vi "+S2C_PCIe7841_Process.vi"(8 "Error In":errorcluster) -> (0 "Error Out":errorcluster)   [LabVIEW 2015]
uses:
  VIs/Typedefs/S2C_PCIe7841_Type_Conn0.ctl
  VIs/Typedefs/S2C_PCIe7841_Type_Conn1.ctl
  VIs/Typedefs/S2C_PCIe7841_Type_Conn2.ctl
  VIs/Typedefs/S2C_PCIe7841_Type_Conn0Write.ctl
  VIs/Typedefs/S2C_PCIe7841_Type_Conn1Write.ctl
  VIs/Typedefs/S2C_PCIe7841_Type_Conn2Write.ctl
  VIs/S2C_PCIe7841_Proc_Globals.vi
panel:
  out "Init":bool
  out "Err":bool
  in  "Clear":bool
  out "Exit":bool
  in  "LogDepth":u32=10 caption="Log Depth"
  in  "CtrlTab":T1(tab)
  in  "P1":T2={"Conn0"={"Port 0"={"LxfIpapPower"=TRUE, "LxfAinDiffSelect"=FALSE, "LxfSpare"=FALSE, "VlacSafeIntLock"=FALSE, "VlacPosDiffNi"=FALSE, "VlacNegDiffNi"=FALSE, "Audio1"=FALSE, "Audio2"=FALSE, "P0_Send"=FALSE, "P0_Size"=FALSE, "P0_State"=FALSE}, "Port 1"={"Audio3"=TRUE, "PalletId1Bcd1"=FALSE, "PalletId1Bcd2"=FALSE, "PalletId1Bcd4"=FALSE, "PalletId1Bcd8"=FALSE, "PalletId2Bcd1"=FALSE, "PalletId2Bcd2"=FALSE, "PalletIdLoopback"=FALSE, "P1_Send"=FALSE, "P1_Size"=FALSE, "P1_State"=FALSE}, "P1C1Exe"=FALSE}}
  in  "P2":T3={"Conn1"={"Port 0"={"MeasM1ErgInp"=TRUE, "MeasLoadBxAct"=FALSE, "MeasLoadBxNeu"=FALSE, "MeasDiffProbAct"=FALSE, "MeasDiffProbNeu"=FALSE, "MeasRemReturn"=FALSE, "MeasBipReturn"=FALSE, "MeasM2ErgInp"=FALSE, "P3_Send"=FALSE, "P3_Size"=FALSE, "P3_State"=FALSE}, "Port 1"={"MeasBipErgInp"=TRUE, "MeasLxBiM1ErgInp"=FALSE, "MeasLxBipM1Rtn"=FALSE, "MeasLxfLigRtn"=FALSE, "MeasLxfLigErgInp"=FALSE, "MeasGndResRtn"=FALSE, "MeasGndResAct"=FALSE, "MeasHomerRelay"=FALSE, "P1_Send"=FALSE, "P1_Size"=FALSE, "P1_State"=FALSE}, "Port 2"={"RemRelayCtrl1"=TRUE, "RemRelayCtrl2"=FALSE, "RemSpare"=FALSE, "RemLoopback"=FALSE, "Mono1Cut_HS"=FALSE, "Mono1Coag_HS"=FALSE, "Mono1Spare"=FALSE, "Mono1Loopback"=FALSE, "P2_Send"=FALSE, "P2_Size"=FALSE, "P2_State"=FALSE}, "Port 3"={"Mono2Cut_HS"=TRUE, "Mono2Coag_HS"=FALSE, "Mono2Spare"=FALSE, "Mono2Loopback"=FALSE, "SmokeBip_HS"=FALSE, "SmokeEvac2"=FALSE, "SmokeEvac1"=FALSE, "SmokeEvacLB"=FALSE, "P3_Send"=FALSE, "P3_Size"=FALSE, "P3_State"=FALSE}, "Port 4"={"MeasSpare"=TRUE, "MeasHomerRtn"=FALSE, "MeasHomerDrive"=FALSE, "MeasLoopback"=FALSE, "VlacDcPwrEnbl"=FALSE, "VlacUartTxNi"=FALSE, "VlacUartRxNi"=FALSE, "VlacRmtPwrNi"=FALSE, "P4_Send"=FALSE, "P4_Size"=FALSE, "P4_State"=FALSE}, "P2C1Exe"=FALSE}}
  in  "P3":T4={"Conn2"={"Port 0"={"TriMono2Mode"=TRUE, "TriMono2Intsy"=FALSE, "TriSliderCtrl"=FALSE, "TriSliderIntsyAdd"=FALSE, "TriSliderIntsyA1"=FALSE, "TriSliderIntsyA0"=FALSE, "TriMono2Slider3"=FALSE, "TriMono2Slider2"=FALSE, "P0_Send"=FALSE, "P0_Size"=FALSE, "P0_State"=FALSE}, "Port 1"={"TriMono2Slider1"=TRUE, "TriSliderIntsyEnbl"=FALSE, "TriSliderEnbl"=FALSE, "TriSpare"=FALSE, "Free1"=FALSE, "Free2"=FALSE, "Free3"=FALSE, "Free4"=FALSE, "P1_Send"=FALSE, "P1_Size"=FALSE, "P1_State"=FALSE}, "Port 2"={"LxfHsw0Ctrl"=TRUE, "LxfLpapPwr"=FALSE, "LxfHpapEnbl"=FALSE, "LxfS2/L4Select"=FALSE, "LxfD/ASelect"=FALSE, "LxfAIn/OutSelect"=FALSE, "LxfALadPortSel"=FALSE, "LxfS2/L4Do"=FALSE, "P2_Send"=FALSE, "P2_Size"=FALSE, "P2_State"=FALSE}, "Port 3"={"LxfS2/L4Di"=FALSE, "LxfS3/L3Do"=TRUE, "LxfS3/L3Di"=FALSE, "LxfHpapAi"=FALSE, "LxfDEnable"=FALSE, "LxfDA1"=FALSE, "LxfDA0"=FALSE, "LxfUartSelect"=FALSE, "P3_Send"=FALSE, "P3_Size"=FALSE, "P3_State"=FALSE}, "Port 4"={"LxfNegChLoopBk"=TRUE, "LxfPosChLoopBk"=FALSE, "LxfRs485DriveDir"=FALSE, "LxfHsw1Ctrl"=FALSE, "LoadSwitchRsvd1"=FALSE, "LoadSwitchRsvd2"=FALSE, "LoadSwitchRsvd3"=FALSE, "LoadSwitchRsvd4"=FALSE, "P4_Send"=FALSE, "P4_Size"=FALSE, "P4_State"=FALSE}, "P3C1Exe"=FALSE}}
  in  "P4":T5
  in  "P5":T12 {"Digital Write"."Connector" items=["Connector 0", "Connector 1", "Connector 2"]; "Digital Write"."Conn2_Item" items=["TriMono2Mode"=0, "TriMono2Intsy"=1, "TriSliderCtrl"=2, "TriSliderIntsyAdd"=3, "TriSliderIntsyA1"=4, "TriSliderIntsyA0"=5, "TriMono2Slider3"=6, "TriMono2Slider2"=7, "TriMono2Slider1"=8, "TriSliderIntsyEnbl"=9, "TriSliderEnbl"=10, "TriSpare"=11, "Free1"=12, "Free2"=13, "Free3"=14, "Free4"=15, "LxfHsw0Ctrl"=16, "LxfLpapPwr"=17, "LxfHpapEnbl"=18, "LxfS2/L4Select"=19, "LxfD/ASelect"=20, "LxfAIn/OutSelect"=21, "LxfALadPortSel"=22, "LxfS2/L4Do"=23, "LxfS3/L3Do"=25, "LxfHpapAi"=27, "LxfDEnable"=28, "LxfDA1"=29, "LxfDA0"=30, "LxfUartSelect"=31, "LxfNegChLoopBk"=32, "LxfPosChLoopBk"=33, "LxfRs485DriveDir"=34, "LxfHsw1Ctrl"=35, "LoadSwitchRsvd1"=36, "LoadSwitchRsvd2"=37, "LoadSwitchRsvd3"=38, "LoadSwitchRsvd4"=39]; "Digital Write"."Conn1_Item" items=["MeasM1ErgInput"=0, "MeasLoadBxAct"=1, "MeasLoadBxNeu"=2, "MeasDiffProbAct"=3, "MeasDiffProbNeu"=4, "MeasRemReturn"=5, "MeasBipReturn"=6, "MeasM2ErgInp"=7, "MeasBipErgInp"=8, "MeasLxBpM1ErgInp"=9, "MeasLxBipM1Rtn"=10, "MeasLxfLigRtn"=11, "MeasLxfLigErgInp"=12, "MeasGndResRtn"=13, "MeasGndResAct"=14, "MeasHomerRelay"=15, "RemRelayCtrl1"=16, "RemRelayCtrl2"=17, "RemSpare"=18, "Mono1Cut_HS"=20, "Mono1Coag_HS"=21, "Mono1Spare"=22, "Mono2Cut_HS"=24, "Mono2Coag_HS"=25, "Mono2Spare"=26, "SmokeBip_HS"=28, "MeasSpare"=32, "MeasHomerRtn"=33, "VlacDcPwrEnbl"=36, "VlacUartTxNi"=37]; "Digital Write"."Conn0_Item" items=["LxfIpapPower"=0, "LxfAinDiffSelect"=1, "LxfSpare"=2, "Audio1"=6, "Audio2"=7, "Audio3"=8]; "Digital Read"."Connector" items=["Connector 0", "Connector 1", "Connector 2"]; "Digital Read"."Conn2_Item" items=["TriMono2Mode", "TriMono2Intsy", "TriSliderCtrl", "TriSliderIntsyAdd", "TriSliderIntsyA1", "TriSliderIntsyA0", "TriMono2Slider3", "TriMono2Slider2", "TriMono2Slider1", "TriSliderIntsyEnbl", "TriSliderEnbl", "TriSpare", "Free1", "Free2", "Free3", "Free4", "LxfHsw0Ctrl", "LxfLpapPwr", "LxfHpapEnbl", "LxfS2/L4Select", "LxfD/ASelect", "LxfAIn/OutSelect", "LxfALadPortSel", "LxfS2/L4Do", "LxfS2/L4Di", "LxfS3/L3Do", "LxfS3/L3Di", "LxfHpapAi", "LxfDEnable", "LxfDA1", "LxfDA0", "LxfUartSelect", "LxfNegChLoopBk", "LxfPosChLoopBk", "LxfRs485DriveDir", "LxfHsw1Ctrl", "LoadSwitchRsvd1", "LoadSwitchRsvd2", "LoadSwitchRsvd3", "LoadSwitchRsvd4"]; "Digital Read"."Conn1_Item" items=["MeasM1ErgInput (75kHz)", "MeasLoadBxAct (75kHz)", "MeasLoadBxNeu (75kHz)", "MeasDiffProbAct (75kHz)", "MeasDiffProbNeu (75kHz)", "MeasRemReturn (75kHz)", "MeasBipReturn (75kHz)", "MeasM2ErgInp (75kHz)", "MeasBipErgInp (75kHz)", "MeasLxBpM1ErgInp (75kHz)", "MeasLxBipM1Rtn (75kHz)", "MeasLxfLigRtn (75kHz)", "MeasLxfLigErgInp (75kHz)", "MeasGndResRtn (75kHz)", "MeasGndResAct (75kHz)", "MeasHomerRelay (75kHz)", "RemRelayCtrl1 (75kHz)", "RemRelayCtrl2 (75kHz)", "RemSpare", "RemLoopback", "Mono1Cut_HS (75kHz)", "Mono1Coag_HS (75kHz)", "Mono1Spare", "Mono1Loopback", "Mono2Cut_HS (75kHz)", "Mono2Coag_HS (75kHz)", "Mono2Spare", "Mono2Loopback", "SmokeBip_HS", "SmokeEvac2", "SmokeEvac1", "SmokeEvacLB", "MeasSpare", "MeasHomerRtn", "MeasHomerDrive", "MeasLoopback", "VlacDcPwrEnbl", "VlacUartTxNi", "VlacUartRxNi", "VlacTmtPwrNi"]; "Digital Read"."Conn0_Item" items=["LxfIpapPower", "LxfAinDiffSelect", "LxfSpare", "VlacSafeIntLock", "VlacPosDiffNi", "VlacNegDiffNi", "Audio1", "Audio2", "Audio3", "PalletId1BCD1", "PalletId1BCD2", "PalletId1BCD4", "PalletId1BCD8", "PalletId2BCD1", "PalletId2BCD2", "PalletIdLoopback"]}
  in  "P6":T13 {"Analog Read"."AO7" min=-10.0 max=10.0 format="%#.6g"; "Analog Read"."AO6" min=-10.0 max=10.0 format="%#.6g"; "Analog Read"."AO5" min=-10.0 max=10.0 format="%#.6g"; "Analog Read"."AO4" min=-10.0 max=10.0 format="%#.6g"; "Analog Read"."AO3" min=-10.0 max=10.0 format="%#.6g"; "Analog Read"."AO2" min=-10.0 max=10.0 format="%#.6g"; "Analog Read"."AO1" min=-10.0 max=10.0 format="%#.6g"; "Analog Read"."AO0" min=-10.0 max=10.0 format="%#.6g"; "Analog Read"."AI7" min=-10.0 max=10.0 format="%#.6g"; "Analog Read"."AI6" min=-10.0 max=10.0 format="%#.6g"; "Analog Read"."AI5" min=-10.0 max=10.0 format="%#.6g"; "Analog Read"."AI4" min=-10.0 max=10.0 format="%#.6g"; "Analog Read"."AI3" min=-10.0 max=10.0 format="%#.6g"; "Analog Read"."AI2" min=-10.0 max=10.0 format="%#.6g"; "Analog Read"."AI1" min=-10.0 max=10.0 format="%#.6g"; "Analog Read"."AI0" min=-10.0 max=10.0 format="%#.6g"; "Analog Write"."AO7" min=-10.0 max=10.0 format="%#.6g"; "Analog Write"."AO6" min=-10.0 max=10.0 format="%#.6g"; "Analog Write"."AO5" min=-10.0 max=10.0 format="%#.6g"; "Analog Write"."AO4" min=-10.0 max=10.0 format="%#.6g"; "Analog Write"."AO3" min=-10.0 max=10.0 format="%#.6g"; "Analog Write"."AO2" min=-10.0 max=10.0 format="%#.6g"; "Analog Write"."AO1" min=-10.0 max=10.0 format="%#.6g"; "Analog Write"."AO0" min=-10.0 max=10.0 format="%#.6g"}
  in  "CommLog":string caption="Communication Log"
  # "Main Cluster:\n394x886\n1 = 355x876\n2 = 355x438\n3 = 355x292\n4 = 163x438\n6 = 163x292\n8 = 163x219"
  # "PCIe7841 Driver Panel"
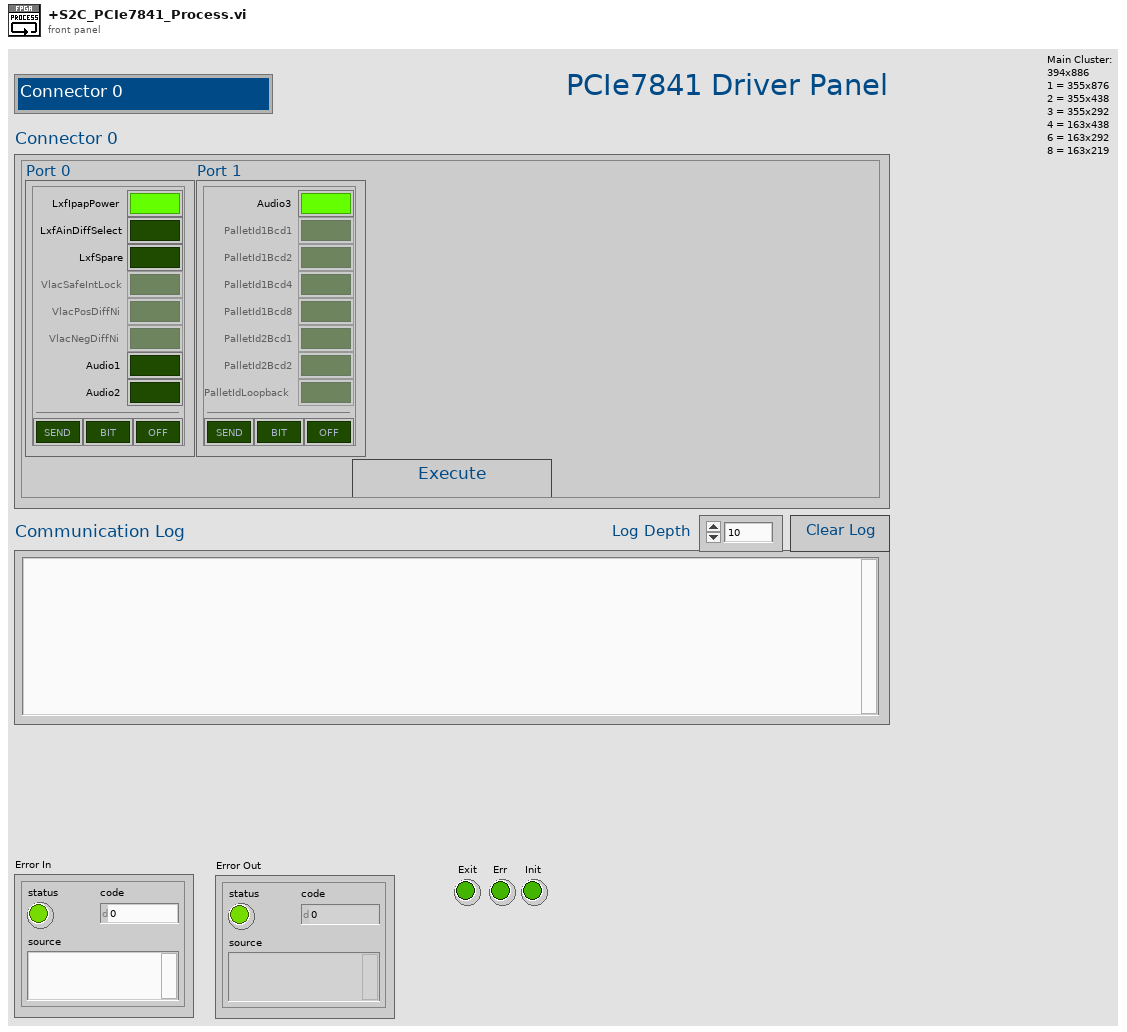
[diagram p1: front panel]
types:
  T1 = enum32{"Connector 0", "Connector 1", "Connector 2", "Status", "Digital IO", "Analog IO"}
  T2 = cluster{"Conn0":cluster{"Port 0":cluster{"LxfIpapPower":bool, "LxfAinDiffSelect":bool, "LxfSpare":bool, "VlacSafeIntLock":bool, "VlacPosDiffNi":bool, "VlacNegDiffNi":bool, "Audio1":bool, "Audio2":bool, "P0_Send":bool, "P0_Size":bool, "P0_State":bool}, "Port 1":cluster{"Audio3":bool, "PalletId1Bcd1":bool, "PalletId1Bcd2":bool, "PalletId1Bcd4":bool, "PalletId1Bcd8":bool, "PalletId2Bcd1":bool, "PalletId2Bcd2":bool, "PalletIdLoopback":bool, "P1_Send":bool, "P1_Size":bool, "P1_State":bool}, "P1C1Exe":bool}}
  T3 = cluster{"Conn1":cluster{"Port 0":cluster{"MeasM1ErgInp":bool, "MeasLoadBxAct":bool, "MeasLoadBxNeu":bool, "MeasDiffProbAct":bool, "MeasDiffProbNeu":bool, "MeasRemReturn":bool, "MeasBipReturn":bool, "MeasM2ErgInp":bool, "P3_Send":bool, "P3_Size":bool, "P3_State":bool}, "Port 1":cluster{"MeasBipErgInp":bool, "MeasLxBiM1ErgInp":bool, "MeasLxBipM1Rtn":bool, "MeasLxfLigRtn":bool, "MeasLxfLigErgInp":bool, "MeasGndResRtn":bool, "MeasGndResAct":bool, "MeasHomerRelay":bool, "P1_Send":bool, "P1_Size":bool, "P1_State":bool}, "Port 2":cluster{"RemRelayCtrl1":bool, "RemRelayCtrl2":bool, "RemSpare":bool, "RemLoopback":bool, "Mono1Cut_HS":bool, "Mono1Coag_HS":bool, "Mono1Spare":bool, "Mono1Loopback":bool, "P2_Send":bool, "P2_Size":bool, "P2_State":bool}, "Port 3":cluster{"Mono2Cut_HS":bool, "Mono2Coag_HS":bool, "Mono2Spare":bool, "Mono2Loopback":bool, "SmokeBip_HS":bool, "SmokeEvac2":bool, "SmokeEvac1":bool, "SmokeEvacLB":bool, "P3_Send":bool, "P3_Size":bool, "P3_State":bool}, "Port 4":cluster{"MeasSpare":bool, "MeasHomerRtn":bool, "MeasHomerDrive":bool, "MeasLoopback":bool, "VlacDcPwrEnbl":bool, "VlacUartTxNi":bool, "VlacUartRxNi":bool, "VlacRmtPwrNi":bool, "P4_Send":bool, "P4_Size":bool, "P4_State":bool}, "P2C1Exe":bool}}
  T4 = cluster{"Conn2":cluster{"Port 0":cluster{"TriMono2Mode":bool, "TriMono2Intsy":bool, "TriSliderCtrl":bool, "TriSliderIntsyAdd":bool, "TriSliderIntsyA1":bool, "TriSliderIntsyA0":bool, "TriMono2Slider3":bool, "TriMono2Slider2":bool, "P0_Send":bool, "P0_Size":bool, "P0_State":bool}, "Port 1":cluster{"TriMono2Slider1":bool, "TriSliderIntsyEnbl":bool, "TriSliderEnbl":bool, "TriSpare":bool, "Free1":bool, "Free2":bool, "Free3":bool, "Free4":bool, "P1_Send":bool, "P1_Size":bool, "P1_State":bool}, "Port 2":cluster{"LxfHsw0Ctrl":bool, "LxfLpapPwr":bool, "LxfHpapEnbl":bool, "LxfS2/L4Select":bool, "LxfD/ASelect":bool, "LxfAIn/OutSelect":bool, "LxfALadPortSel":bool, "LxfS2/L4Do":bool, "P2_Send":bool, "P2_Size":bool, "P2_State":bool}, "Port 3":cluster{"LxfS2/L4Di":bool, "LxfS3/L3Do":bool, "LxfS3/L3Di":bool, "LxfHpapAi":bool, "LxfDEnable":bool, "LxfDA1":bool, "LxfDA0":bool, "LxfUartSelect":bool, "P3_Send":bool, "P3_Size":bool, "P3_State":bool}, "Port 4":cluster{"LxfNegChLoopBk":bool, "LxfPosChLoopBk":bool, "LxfRs485DriveDir":bool, "LxfHsw1Ctrl":bool, "LoadSwitchRsvd1":bool, "LoadSwitchRsvd2":bool, "LoadSwitchRsvd3":bool, "LoadSwitchRsvd4":bool, "P4_Send":bool, "P4_Size":bool, "P4_State":bool}, "P3C1Exe":bool}}
  T5 = cluster{"Status":cluster{"P4C1Exe":bool, "Stat0":cluster{"Port 0":cluster{"B0":bool, "B1":bool, "B2":bool, "B3":bool, "B4":bool, "B5":bool, "B6":bool, "B7":bool}, "Port 1":cluster{"B0":bool, "B1":bool, "B2":bool, "B3":bool, "B4":bool, "B5":bool, "B6":bool, "B7":bool}}, "Stat1":cluster{"Port 0":cluster{"B0":bool, "B1":bool, "B2":bool, "B3":bool, "B4":bool, "B5":bool, "B6":bool, "B7":bool}, "Port 1":cluster{"B0":bool, "B1":bool, "B2":bool, "B3":bool, "B4":bool, "B5":bool, "B6":bool, "B7":bool}, "Port 2":cluster{"B0":bool, "B1":bool, "B2":bool, "B3":bool, "B4":bool, "B5":bool, "B6":bool, "B7":bool}, "Port 3":cluster{"B0":bool, "B1":bool, "B2":bool, "B3":bool, "B4":bool, "B5":bool, "B6":bool, "B7":bool}, "Port 4":cluster{"B0":bool, "B1":bool, "B2":bool, "B3":bool, "B4":bool, "B5":bool, "B6":bool, "B7":bool}}, "Stat2":cluster{"Port 0":cluster{"B0":bool, "B1":bool, "B2":bool, "B3":bool, "B4":bool, "B5":bool, "B6":bool, "B7":bool}, "Port 1":cluster{"B0":bool, "B1":bool, "B2":bool, "B3":bool, "B4":bool, "B5":bool, "B6":bool, "B7":bool}, "Port 2":cluster{"B0":bool, "B1":bool, "B2":bool, "B3":bool, "B4":bool, "B5":bool, "B6":bool, "B7":bool}, "Port 3":cluster{"B0":bool, "B1":bool, "B2":bool, "B3":bool, "B4":bool, "B5":bool, "B6":bool, "B7":bool}, "Port 4":cluster{"B0":bool, "B1":bool, "B2":bool, "B3":bool, "B4":bool, "B5":bool, "B6":bool, "B7":bool}}}}
  T6 = typedef "S2C_PCIe7841_Type_Conn0.ctl" = u16
  T7 = typedef "S2C_PCIe7841_Type_Conn1.ctl" = u16
  T8 = typedef "S2C_PCIe7841_Type_Conn2.ctl" = u16
  T9 = typedef "S2C_PCIe7841_Type_Conn0Write.ctl" = u16
  T10 = typedef "S2C_PCIe7841_Type_Conn1Write.ctl" = u16
  T11 = typedef "S2C_PCIe7841_Type_Conn2Write.ctl" = u16
  T12 = cluster{"Digital Read":cluster{"P5C2Exe":bool, "Conn0_Item":T6, "Conn1_Item":T7, "Conn2_Item":T8, "Connector":u16, "StateOut":bool}, "Digital Write":cluster{"Connector":u16, "Conn0_Item":T9, "Conn1_Item":T10, "Conn2_Item":T11, "StateIn":bool, "P5C1Exe":bool}}
  T13 = cluster{"Analog Write":cluster{"AO0":dbl, "AO0_Send":bool, "AO1":dbl, "AO1_Send":bool, "AO2":dbl, "AO2_Send":bool, "AO3":dbl, "AO3_Send":bool, "AO4":dbl, "AO4_Send":bool, "AO5":dbl, "AO5_Send":bool, "AO6":dbl, "AO6_Send":bool, "AO7":dbl, "AO7_Send":bool, "P6C1Exe":bool}, "Analog Read":cluster{"AI0":dbl, "AI1":dbl, "AI2":dbl, "AI3":dbl, "AI4":dbl, "AI5":dbl, "AI6":dbl, "AI7":dbl, "AO0":dbl, "AO1":dbl, "AO2":dbl, "AO3":dbl, "AO4":dbl, "AO5":dbl, "AO6":dbl, "AO7":dbl, "P6C2Exe":bool}}
  T14 = cluster{"Caller-Q":refnum<queue>, "Command":string, "Return":string, "Data":variant, "Timeout":dbl}
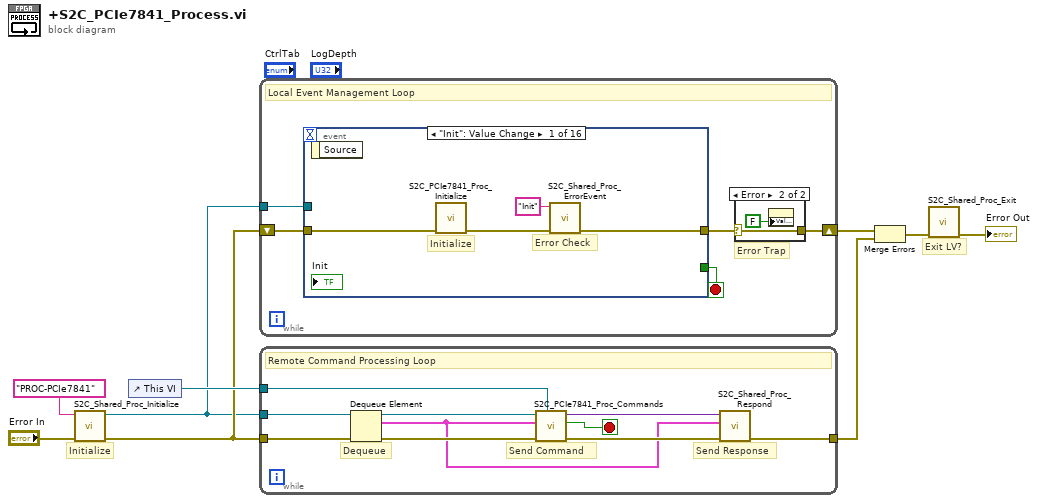
[diagram p0: block diagram]
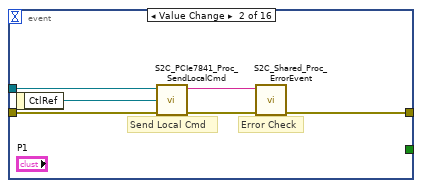
[diagram p3: hidden frame]
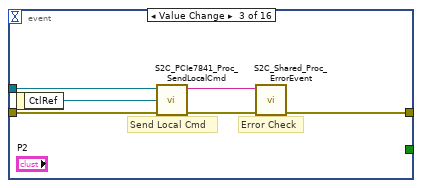
[diagram p4: hidden frame]
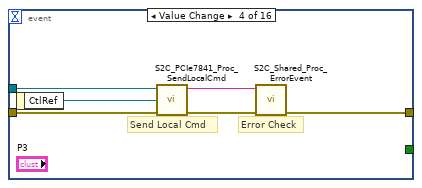
[diagram p5: hidden frame]
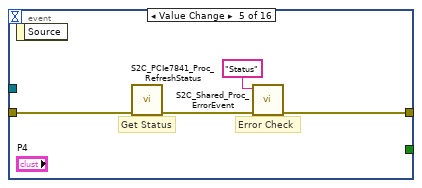
[diagram p6: hidden frame]
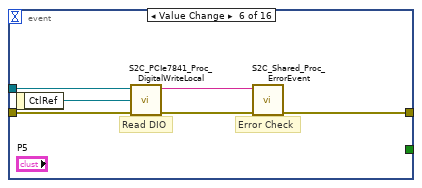
[diagram p7: hidden frame]
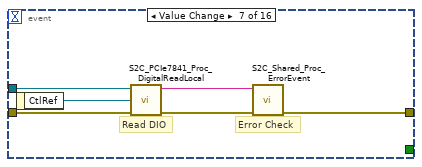
[diagram p8: hidden frame]
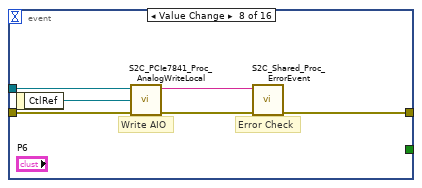
[diagram p9: hidden frame]
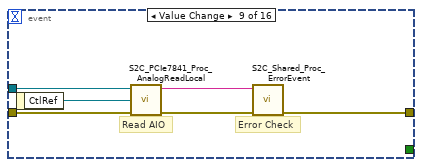
[diagram p10: hidden frame]
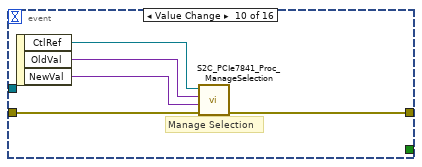
[diagram p11: hidden frame]
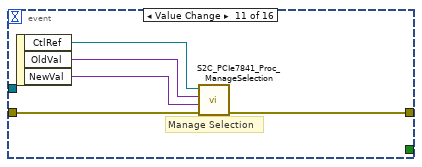
[diagram p12: hidden frame]
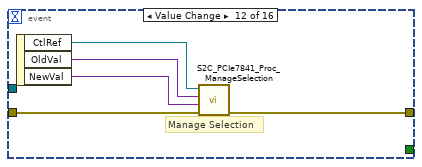
[diagram p13: hidden frame]
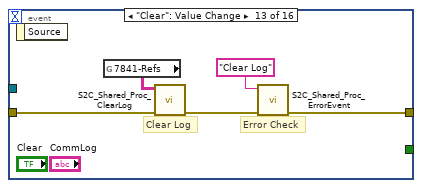
[diagram p14: hidden frame]
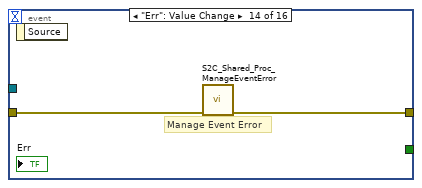
[diagram p15: hidden frame]
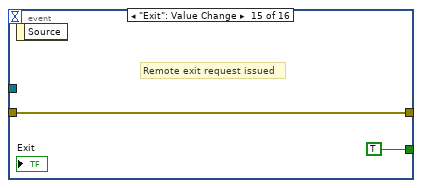
[diagram p16: hidden frame]
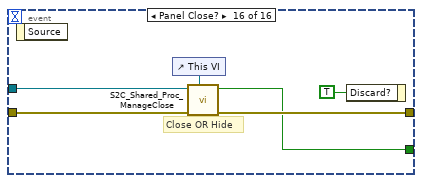
[diagram p17: hidden frame]
diagram:
  # "Exit LV?"
  # "Initialize"
  n1 = call "S2C_Shared_Proc_Initialize.vi"("Error In"="Error In", "Q-Name"="PROC-PCIe7841" ("name (unnamed)")) -> ("Error Out"=w4:errorcluster, "Q-Ref"=w1:refnum<queue>)  [unwired: 8 in]
  n2 = control-ref of="This VI"() -> (w5:refnum<vi>)
  n3 = while {
    tunnel: w1 -> [w13]
    shift-right: [w10] -> w7
    shift-left: w4 -> [w14]
    stop <- w12 stop-if-true
    # "Error Trap"
    # "Local Event Management Loop"
    n4 = event shown="[0] \"Init\": Value Change" {
      selector: _ -> [_ _ _ _ _ _ _ _ _ _ _ _ _ _ _ _]
      dyn-events: _ -> [_ _ _ _ _ _ _ _ _ _ _ _ _ _ _ _]
      timeout: _ -> [_ _ _ _ _ _ _ _ _ _ _ _ _ _ _ _]
      tunnel: w14 -> [w21 w27 w33 w39 w42 w48 w54 w60 w66 w71 w76 w81 w87 w89 w91 w96]
      tunnel: w13 -> [_ w26 w32 w38 _ w46 w52 w58 w64 _ _ _ _ _ _ w94]
      tunnel: [w18 w23 w29 w35 w43 w49 w55 w61 w67 w72 w77 w82 w85 w88 w91 w95] -> w11
      tunnel: [_ _ _ _ _ _ _ _ _ _ _ _ _ _ TRUE ("Discard?") w93] -> w12
      event "Init": Value Change {
        # "Error Check"
        # "Initialize"
        n5 = event-data() -> ()  [unwired: 1 in, 1 out]
        n6 = call "S2C_PCIe7841_Proc_Initialize.vi"("Error In"=w21) -> ("Error Out"=w19:errorcluster)  [unwired: 10 in]
        n7 = call "S2C_Shared_Proc_ErrorEvent.vi"("Error In"=w19, "Command"="Init") -> ("Error Out"=w18:errorcluster)  [unwired: 9 in]
      }
      event "P1.Conn0.P1C1Exe": Value Change {
        # "Error Check"
        # "Send Local Cmd"
        n8 = event-data() -> ("CtlRef"=w25:refnum<vi>)  [unwired: 1 in]
        n9 = call "S2C_PCIe7841_Proc_SendLocalCmd.vi"("Error In"=w27, "ExeRef"=w25, "Q-Ref"=w26) -> ("Error Out"=w24:errorcluster, "Command"=w22:string)  [unwired: 7 in]
        n10 = call "S2C_Shared_Proc_ErrorEvent.vi"("Error In"=w24, "Command"=w22) -> ("Error Out"=w23:errorcluster)  [unwired: 9 in]
      }
      event "P2.Conn1.P2C1Exe": Value Change {
        # "Error Check"
        # "Send Local Cmd"
        n11 = event-data() -> ("CtlRef"=w31:refnum<vi>)  [unwired: 1 in]
        n12 = call "S2C_PCIe7841_Proc_SendLocalCmd.vi"("Error In"=w33, "ExeRef"=w31, "Q-Ref"=w32) -> ("Error Out"=w30:errorcluster, "Command"=w28:string)  [unwired: 7 in]
        n13 = call "S2C_Shared_Proc_ErrorEvent.vi"("Error In"=w30, "Command"=w28) -> ("Error Out"=w29:errorcluster)  [unwired: 9 in]
      }
      event "P3.Conn2.P3C1Exe": Value Change {
        # "Error Check"
        # "Send Local Cmd"
        n14 = event-data() -> ("CtlRef"=w37:refnum<vi>)  [unwired: 1 in]
        n15 = call "S2C_PCIe7841_Proc_SendLocalCmd.vi"("Error In"=w39, "ExeRef"=w37, "Q-Ref"=w38) -> ("Error Out"=w36:errorcluster, "Command"=w34:string)  [unwired: 7 in]
        n16 = call "S2C_Shared_Proc_ErrorEvent.vi"("Error In"=w36, "Command"=w34) -> ("Error Out"=w35:errorcluster)  [unwired: 9 in]
      }
      event "P4.Status.P4C1Exe": Value Change {
        # "Get Status"
        # "Error Check"
        n17 = event-data() -> ()  [unwired: 1 in, 1 out]
        n18 = call "S2C_PCIe7841_Proc_RefreshStatus.vi"("Error In"=w42) -> ("Error Out"=w41:errorcluster)  [unwired: 10 in]
        n19 = call "S2C_Shared_Proc_ErrorEvent.vi"("Error In"=w41, "Command"="Status") -> ("Error Out"=w43:errorcluster)  [unwired: 9 in]
      }
      event "P5.Digital Write.P5C1Exe": Value Change {
        # "Read DIO"
        # "Error Check"
        n20 = event-data() -> ("CtlRef"=w45:refnum<vi>)  [unwired: 1 in]
        n21 = call "S2C_PCIe7841_Proc_DigitalWriteLocal.vi"("Error In"=w48, "ExeRef"=w45, "Q-Ref"=w46) -> ("Error Out"=w47:errorcluster, "Command"=w44:string)  [unwired: 7 in]
        n22 = call "S2C_Shared_Proc_ErrorEvent.vi"("Error In"=w47, "Command"=w44) -> ("Error Out"=w49:errorcluster)  [unwired: 9 in]
      }
      event "P5.Digital Read.P5C2Exe": Value Change {
        # "Read DIO"
        # "Error Check"
        n23 = event-data() -> ("CtlRef"=w51:refnum<vi>)  [unwired: 1 in]
        n24 = call "S2C_PCIe7841_Proc_DigitalReadLocal.vi"("Error In"=w54, "ExeRef"=w51, "Q-Ref"=w52) -> ("Error Out"=w53:errorcluster, "Command"=w50:string)  [unwired: 7 in]
        n25 = call "S2C_Shared_Proc_ErrorEvent.vi"("Error In"=w53, "Command"=w50) -> ("Error Out"=w55:errorcluster)  [unwired: 9 in]
      }
      event "P6.Analog Write.P6C1Exe": Value Change {
        # "Write AIO"
        # "Error Check"
        n26 = event-data() -> ("CtlRef"=w57:refnum<vi>)  [unwired: 1 in]
        n27 = call "S2C_PCIe7841_Proc_AnalogWriteLocal.vi"("Error In"=w60, "ExeRef"=w57, "Q-Ref"=w58) -> ("Error Out"=w59:errorcluster, "Command"=w56:string)  [unwired: 7 in]
        n28 = call "S2C_Shared_Proc_ErrorEvent.vi"("Error In"=w59, "Command"=w56) -> ("Error Out"=w61:errorcluster)  [unwired: 9 in]
      }
      event "P6.Analog Read.P6C2Exe": Value Change {
        # "Read AIO"
        # "Error Check"
        n29 = event-data() -> ("CtlRef"=w63:refnum<vi>)  [unwired: 1 in]
        n30 = call "S2C_PCIe7841_Proc_AnalogReadLocal.vi"("Error In"=w66, "ExeRef"=w63, "Q-Ref"=w64) -> ("Error Out"=w65:errorcluster, "Command"=w62:string)  [unwired: 7 in]
        n31 = call "S2C_Shared_Proc_ErrorEvent.vi"("Error In"=w65, "Command"=w62) -> ("Error Out"=w67:errorcluster)  [unwired: 9 in]
      }
      event "P1.Conn0.Port 0", "P1.Conn0.Port 1": Value Change {
        # "Manage Selection"
        n32 = event-data() -> ("CtlRef"=w68:refnum<vi>, "OldVal"=w69:variant, "NewVal"=w70:variant)  [unwired: 1 in]
        n33 = call "S2C_PCIe7841_Proc_ManageSelection.vi"("Error In"=w71, "NewValue"=w70, "OldValue"=w69, "CtlRef"=w68) -> ("Error Out"=w72:errorcluster)  [unwired: 7 in]
      }
      event "P2.Conn1.Port 0", "P2.Conn1.Port 1", "P2.Conn1.Port 2", "P2.Conn1.Port 3", "P2.Conn1.Port 4": Value Change {
        # "Manage Selection"
        n34 = event-data() -> ("CtlRef"=w73:refnum<vi>, "OldVal"=w74:variant, "NewVal"=w75:variant)  [unwired: 1 in]
        n35 = call "S2C_PCIe7841_Proc_ManageSelection.vi"("Error In"=w76, "NewValue"=w75, "OldValue"=w74, "CtlRef"=w73) -> ("Error Out"=w77:errorcluster)  [unwired: 7 in]
      }
      event "P3.Conn2.Port 0", "P3.Conn2.Port 1", "P3.Conn2.Port 2", "P3.Conn2.Port 3", "P3.Conn2.Port 4": Value Change {
        # "Manage Selection"
        n36 = event-data() -> ("CtlRef"=w78:refnum<vi>, "OldVal"=w79:variant, "NewVal"=w80:variant)  [unwired: 1 in]
        n37 = call "S2C_PCIe7841_Proc_ManageSelection.vi"("Error In"=w81, "NewValue"=w80, "OldValue"=w79, "CtlRef"=w78) -> ("Error Out"=w82:errorcluster)  [unwired: 7 in]
      }
      event "Clear": Value Change {
        # "Error Check"
        # "Clear Log"
        n38 = event-data() -> ()  [unwired: 1 in, 1 out]
        n39 = global read "S2C_PCIe7841_Proc_Globals.vi" "7841-Refs"() -> (w83:string[][])
        n40 = call "S2C_Shared_Proc_ClearLog.vi"("Error In"=w87, "Refs"=w83) -> ("Error Out"=w86:errorcluster)  [unwired: 9 in]
        n41 = call "S2C_Shared_Proc_ErrorEvent.vi"("Error In"=w86, "Command"="Clear Log") -> ("Error Out"=w85:errorcluster)  [unwired: 9 in]
      }
      event "Err": Value Change {
        # "Manage Event Error"
        n42 = event-data() -> ()  [unwired: 1 in, 1 out]
        n43 = call "S2C_Shared_Proc_ManageEventError.vi"("Error In"=w89) -> ("Error Out"=w88:errorcluster)  [unwired: 10 in]
      }
      event "Exit": Value Change {
        # "Remote exit request issued"
        n44 = event-data() -> ()  [unwired: 1 in, 1 out]
      }
      event Panel Close? {
        # "Close OR Hide"
        n45 = event-data() -> ()  [unwired: 1 in, 1 out]
        n46 = control-ref of="This VI"() -> (w92:refnum<vi>)
        n47 = call "S2C_Shared_Proc_ManageClose.vi"("VI_Ref"=w92, "Error In"=w96, "Q-Ref"=w94) -> ("Error Out"=w95:errorcluster, "Exit?"=w93:bool)  [unwired: 7 in]
        n48 = event-data("Discard?"=TRUE) -> ()  [unwired: 1 in, 1 out]
      }
    }
    n49 = case shown="Error" w11 {
      selector: w11 -> [w15 w17]
      tunnel: [w15 w17] -> w10
      frame No Error {
      }
      frame Error {
        n50 = property on="Err" class="Bool (strict)"("Val(Sgnl)"=FALSE ("Value (Signaling)")) -> ()  [unwired: 2 in, 2 out]
      }
    }
  }
  n51 = while {
    tunnel: w1 -> [w98]
    tunnel: w5 -> [w102]
    tunnel: w4 -> [w107]
    tunnel: [w101] -> w6
    stop <- w103 stop-if-true
    # "Send Response"
    # "Send Command"
    # "Dequeue"
    # "Remote Command Processing Loop"
    n52 = Dequeue Element(queue=w98, error in (no error)=w107) -> (queue out=w100:refnum<queue>, element=w99:T14, error out=w106:errorcluster)  [unwired: 1 in, 1 out]
    n53 = call "S2C_PCIe7841_Proc_Commands.vi"("VI_Ref"=w102, "Error In"=w106, "Settings"=w99, "Q-Ref"=w100) -> ("Error Out"=w104:errorcluster, "Stop?"=w103:bool, "Response"=w105:variant)  [unwired: 5 in]
    n54 = call "S2C_Shared_Proc_Respond.vi"("Error In"=w104, "Settings"=w99, "Response"=w105) -> ("Error Out"=w101:errorcluster)  [unwired: 8 in]
  }
  n55 = Merge Errors(w7, w6) -> (w3:errorcluster)
  n56 = call "S2C_Shared_Proc_Exit.vi"("Error In"=w3) -> ("Error Out"=→"Error Out":errorcluster)  [unwired: 10 in]
